vi "Event-driven Scenario (Event Method).vi"() -> ()   [LabVIEW 2014]
panel:
  out "波形图":dynamicdata(graph)
  in  "采集数据":bool
  out "温度（华氏度）":dbl=32.0
  in  "温度（摄氏度）":dbl
  in  "时间检查":bool
  out "当前时间":timestamp
  in  "停止":bool
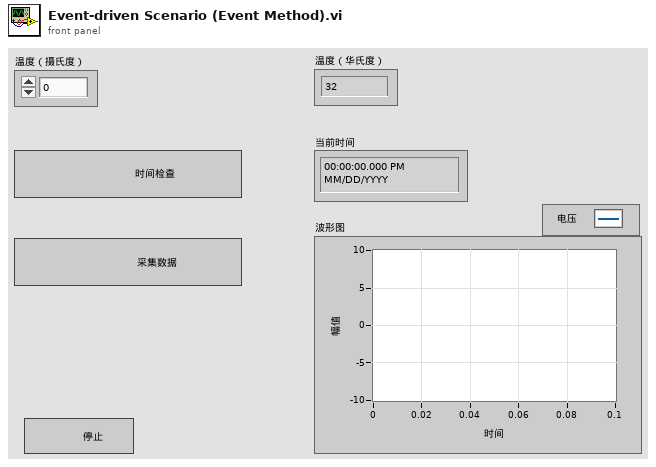
[diagram p1: front panel]
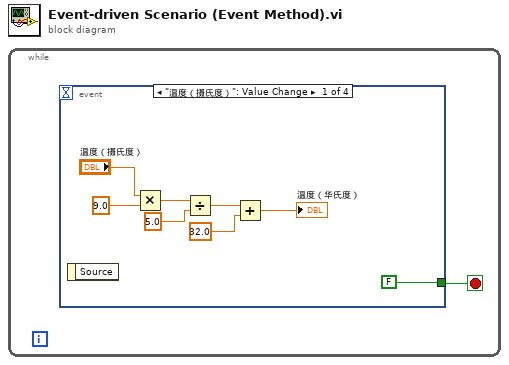
[diagram p0: block diagram]
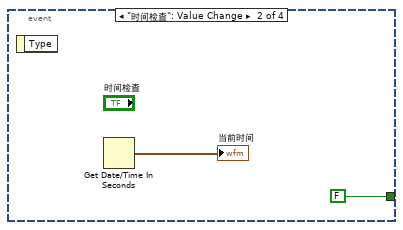
[diagram p2: hidden frame]
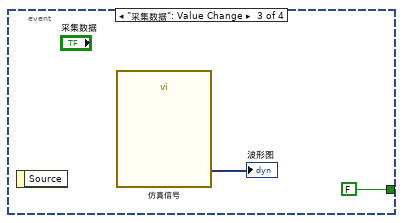
[diagram p3: hidden frame]
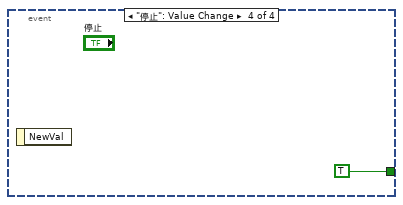
[diagram p4: hidden frame]
diagram:
  n1 = while {
    stop <- w1 stop-if-true
    n2 = event shown="[0] \"温度（摄氏度）\": Value Change" {
      selector: _ -> [_ _ _ _]
      dyn-events: _ -> [_ _ _ _]
      timeout: _ -> [_ _ _ _]
      tunnel: [FALSE FALSE FALSE TRUE] -> w1
      event "温度（摄氏度）": Value Change {
        n3 = event-data() -> ()  [unwired: 1 in, 1 out]
        n4 = Multiply(x="温度（摄氏度）", y=9.0) -> (x*y=w7:dbl)
        n5 = Divide(x=w7, y=5.0) -> (x/y=w5:dbl)
        n6 = Add(x=w5, y=32.0) -> (x+y=→"温度（华氏度）":dbl)
      }
      event "时间检查": Value Change {
        n7 = event-data() -> ()  [unwired: 1 in, 1 out]
        n8 = Get Date/Time In Seconds() -> (seconds since 1Jan1904=→"当前时间":timestamp)
      }
      event "采集数据": Value Change {
        n9 = event-data() -> ()  [unwired: 1 in, 1 out]
        n10 = call "仿真信号"() -> ("Sine with Uniform Noise"=→"波形图":dynamicdata)  [unwired: 14 in, 1 out]
      }
      event "停止": Value Change {
        n11 = event-data() -> ()  [unwired: 1 in, 1 out]
      }
    }
  }
